vi "ThrottleToMaintainCargoInIntake.vi"(10 "Current above threshold?":bool, 11 "Cargo's intended throttle":dbl) -> (3 "Modified Throttle":dbl)   [LabVIEW 2018]
panel:
  in  "How Much To Pull to keep ball in":dbl=0.2
  # "ASSUMES POSITIVE IS IN"
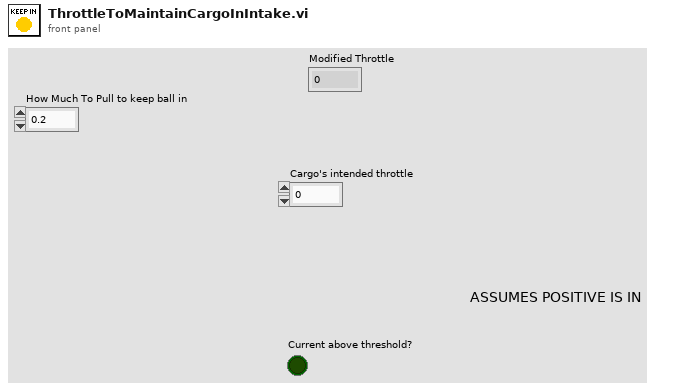
[diagram p1: front panel]
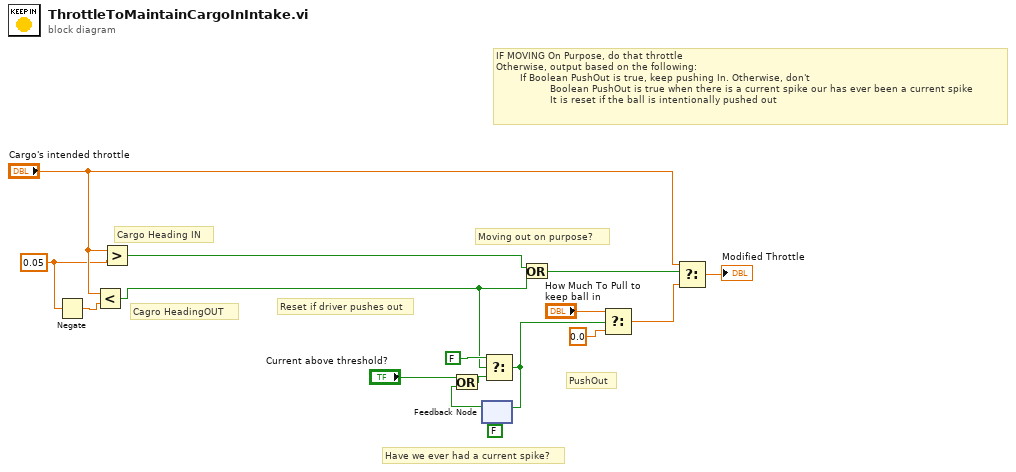
[diagram p0: block diagram]
diagram:
  w3 = 0.05
  # "Cagro HeadingOUT"
  # "Cargo Heading IN"
  # "Have we ever had a current spike?"
  # "Reset if driver pushes out"
  # "PushOut"
  # "Moving out on purpose?"
  # "IF MOVING On Purpose, do that throttle\nOtherwise, output based on the following:\n        If Boolean PushOut is true, keep pushing In. Otherwise, don't\n                  Boolean PushOut is true when there is a current spike our has ever been a current spike\n                  It is reset if the ball is intentionally pushed out"
  n1 = Negate(x=w3) -> (-x=w4:dbl)
  n2 = Less?(x="Cargo's intended throttle", y=w4) -> (x < y?=w1:bool)
  n3 = Greater?(x="Cargo's intended throttle", y=w3) -> (0:w2:bool)
  n4 = feedback #1(FALSE) -> (w13:bool)
  n5 = Or(x="Current above threshold?", y=w13) -> (x .or. y?=w14:bool)
  n6 = Select(t=FALSE, s=w1, f=w14) -> (s? t:f=w8:bool)
  n7 = feedback-in #1(w8) -> ()
  n8 = Or(x=w2, y=w1) -> (x .or. y?=w16:bool)
  n9 = Select(t="How Much To Pull to keep ball in", s=w8, f=0.0) -> (s? t:f=w10:dbl)
  n10 = Select(t="Cargo's intended throttle", s=w16, f=w10) -> (s? t:f=→"Modified Throttle":dbl)
